vi "DSF.Engine.Sequencer.Start of Cycle.vi"(8 "error in (no error)":errorcluster, 10 "engine iteration":u64, 11 "Sequencer in":refnum<class "DSF.Engine.Sequencer.lvclass">) -> (0 "error out":errorcluster, 3 "Sequencer out":refnum<class "DSF.Engine.Sequencer.lvclass">)   [LabVIEW 2016, in "DSF.Engine.lvlib" / "DSF.Engine.Sequencer.lvclass"]
uses:
  DSF.Engine.Sequencer.lvclass
  Timing/DSF.Engine.Timing.lvclass
  DSF.Engine.Sequencer.Plugin State Data.ctl
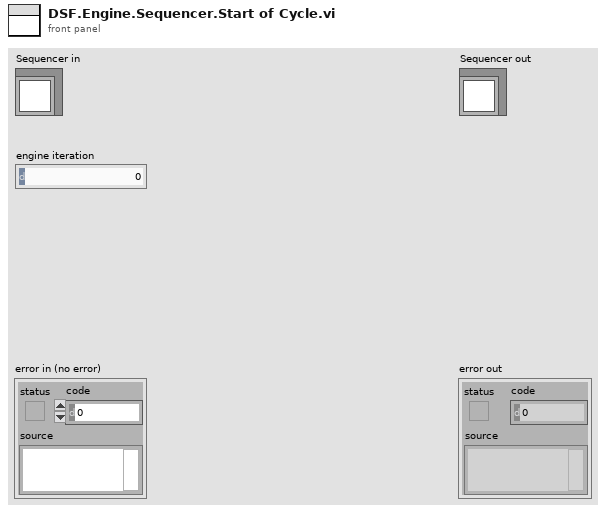
[diagram p1: front panel]
types:
  T1 = typedef "DSF.Engine.lvlib/DSF.Engine.Sequencer.lvclass/DSF.Engine.Sequencer.Plugin State Data.ctl" = cluster{"iteration":u64}
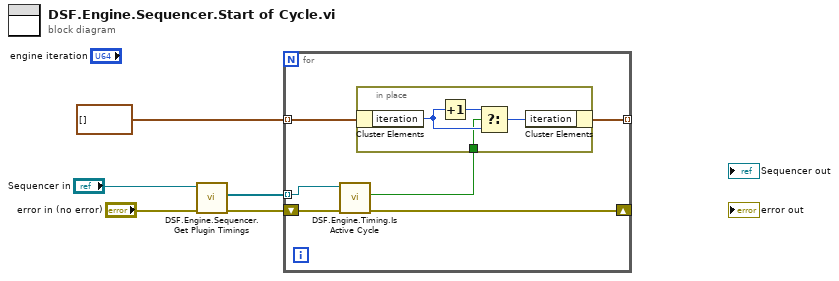
[diagram p0: block diagram]
diagram:
  n1 = call "DSF.Engine.Sequencer.Get Plugin Timings.vi"("error in (no error)"="error in (no error)", "Sequencer in"="Sequencer in") -> ("error out"=w3:errorcluster, "Plugin Timings"=w1:refnum<class "DSF.Engine.Timing.lvclass">[])  [unwired: 7 in, 1 out]
  n2 = for {
    shift-right: [w10] -> _
    shift-left: w3 -> [w11]
    tunnel: T1[] [] ("Array") -> [w9] mode=indexing
    tunnel: [w8] -> _ mode=indexing
    tunnel: w1 -> [w6] mode=indexing
    n3 = call "DSF.Engine.Timing.Is Active Cycle.vi"("error in (no error)"=w11, "Execution Timing in"=w6) -> ("error out"=w10:errorcluster, "active?"=w7:bool)  [unwired: 7 in, 1 out]
    n4 = in-place {
      in-place-border: w7 -> [w14]
      n5 = in-place-cluster #1(w9) -> ("iteration"=w15:u64)
      n6 = Increment(x=w15) -> (x+1=w13:u64)
      n7 = Select(t=w13, s=w14, f=w15) -> (s? t:f=w12:u64)
      n8 = in-place-cluster #1("iteration"=w12) -> (w8:T1)
    }
  }
